vi "From Variant.vi"(8 "Error In":errorcluster, 10 "Variant":variant, 11 "TD Path A In":refnum<class "1D Path.lvclass">) -> (0 "Error Out":errorcluster, 3 "TD Path A Out":refnum<class "1D Path.lvclass">)   [LabVIEW 2020, in "NI_VIAnCFGDataStructure.lvlib" / "1D Path.lvclass"]
doc: "Dynamic dispatch interface for conversion of variant LV data to Tree Data classes."
uses:
  <vilib>/addons/analyzer/VIAnCFGDataStructure/Data Types/Path Array/1D Path.lvclass
  <vilib>/addons/analyzer/VIAnCFGDataStructure/Data Types/Path Array/1D Path.lvclass/1D Path.ctl
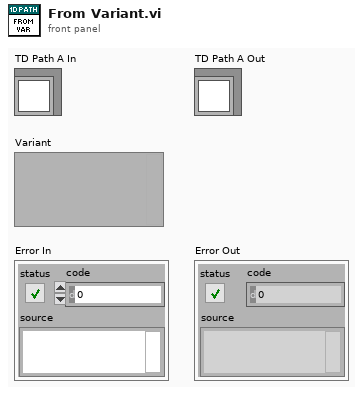
[diagram p1: front panel]
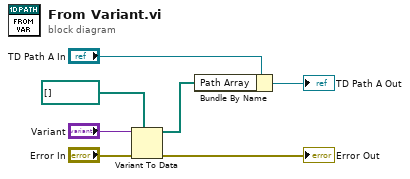
[diagram p0: block diagram]
diagram:
  n1 = Variant To Data(error in="Error In", type=path[] [], Variant="Variant") -> (data=w2:path[], error out=→"Error Out":errorcluster)
  n2 = Bundle By Name(cluster="TD Path A In", "Path Array"=w2) -> (→"TD Path A Out":refnum<class "1D Path.lvclass">)
